vi "IMAQdx Get Image2.vi"(5 "Timeout (ms)":i32=5000, 7 "Buffer Number Mode (Next)":T1, 8 "error in":errorcluster, 9 "Buffer Number In":u32, 10 "Image In":T2, 11 "Session In":T3) -> (0 "error out":errorcluster, 1 "Buffer Number Out":u32, 2 "Image Out":T2, 3 "Session Out":T3)   [LabVIEW 2020, in "NI_Vision_Acquisition_Software.lvlib"]
doc: "Acquires the specified frame into <B>Image Out</B>. Call this VI only after calling the IMAQdx Configure Acquisition VI. If the image type does not match the video format of the camera, this VI changes the image type to a suitable format."
uses:
  NI_Vision_Acquisition_Software.lvlib
  IMAQdx.ctl
  IMAQ Image.ctl
  IMAQdx Buffer Number Mode.ctl
  niimaqdx.dll
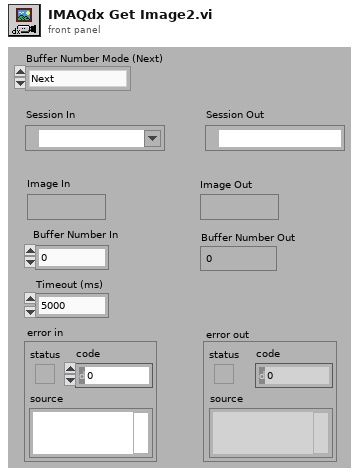
[diagram p1: front panel]
types:
  T1 = typedef "NI_Vision_Acquisition_Software.lvlib/IMAQdx Buffer Number Mode.ctl" = enum32{"Next", "Last", "Buffer Number", "Every", "Last New"}
  T2 = typedef "IMAQ Image.ctl" = refnum<image>
  T3 = typedef "IMAQdx.ctl" = refnum<k21>
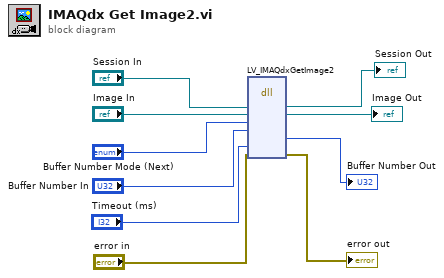
[diagram p0: block diagram]
diagram:
  n1 = dll-call lib="niimaqdx.dll" fn="LV_IMAQdxGetImage2"("refnum"="Session In", "image"="Image In", "mode"="Buffer Number Mode (Next)", "bufferNumberDesired"="Buffer Number In", "timeoutMs"="Timeout (ms)", "error"="error in") -> ("refnum"=→"Session Out":T3, "image"=→"Image Out":T2, "bufferNumberActual"=→"Buffer Number Out":u32, "error"=→"error out":errorcluster)  [unwired: 8 in, 2 out]
